vi "recursively populate tree ctl.vi"(8 "error in (no error)":errorcluster, 10 "Object path":string="IndivITX/Test1/SA03008N.20190801.000000.itx", 11 "tree ctl ref":refnum<vi>) -> (0 "error out":errorcluster, 3 "reference out":refnum<vi>)   [LabVIEW 2019, in "LV-Data.S3.lvclass"]
uses:
  LV-Data.S3.lvclass
panel:
  in  "Tree":string(tree)
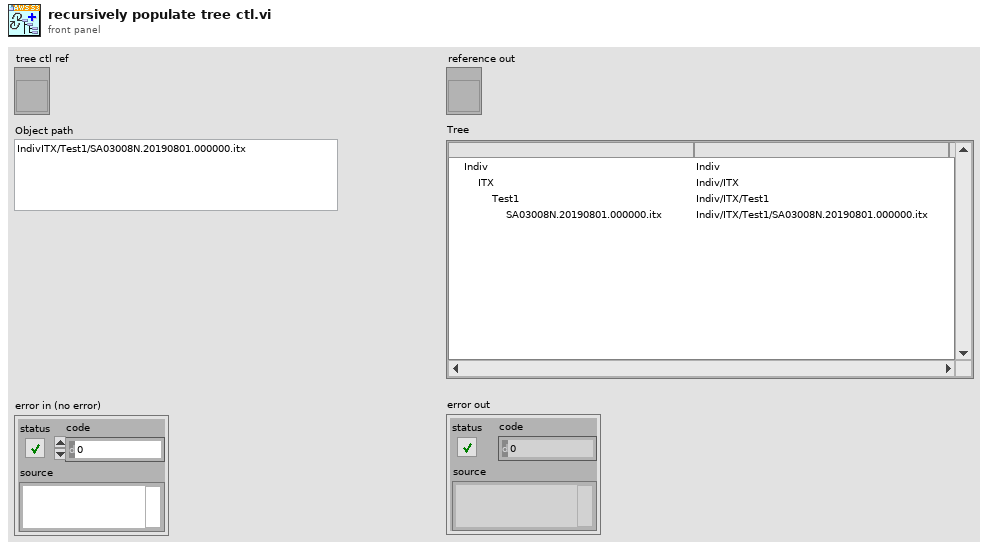
[diagram p1: front panel]
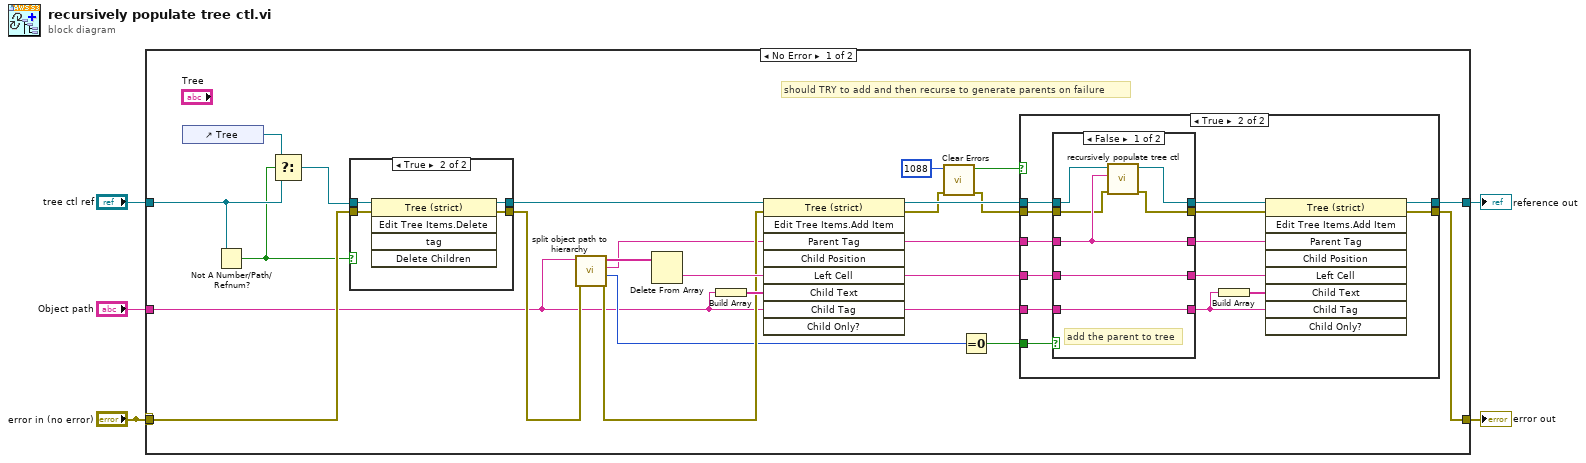
[diagram p0: block diagram]
diagram:
  n1 = case shown="No Error" "error in (no error)" {
    selector: "error in (no error)" -> [_ w62]
    tunnel: [w17 w62] -> w5
    tunnel: [w23 w63] -> w4
    tunnel: "Object path" -> [w8 _]
    tunnel: "tree ctl ref" -> [w7 w63]
    tunnel: "error in (no error)" -> [w10 _]
    frame No Error {
      # "should TRY to add and then recurse to generate parents on failure"
      n2 = control-ref of="Tree"() -> (w18:refnum<vi>)
      n3 = Not A Number/Path/Refnum?(number/path/refnum=w7) -> (NaN/Path/Refnum?=w6:bool)
      n4 = Select(t=w18, s=w6, f=w7) -> (s? t:f=w12:refnum<vi>)
      n5 = case shown="True" w6 {
        tunnel: w12 -> [w29 w33]
        tunnel: [w29 w32] -> w11
        tunnel: w10 -> [w28 w31]
        tunnel: [w28 w30] -> w9
        frame False {
        }
        frame True {
          n6 = invoke class="Tree (strict)" method="Edit Tree Items.Delete"(reference=w33, error in=w31) -> (reference out=w32:refnum<vi>, error out=w30:errorcluster)  [unwired: 3 in, 3 out]
        }
      }
      n7 = call "split object path to hierarchy.vi"("error in (no error)"=w9, "Object path"=w8) -> ("error out"=w19:errorcluster, "layers"=w14:i32, "parent path"=w13:string, "hierarchy"=w21:string[])  [unwired: 6 in]
      n8 = Delete From Array(array=w21) -> (deleted portion=w20:string)  [unwired: 2 in, 1 out]
      n9 = Build Array(w8) -> (w26:string[])
      n10 = invoke on="Invoke Node" class="Tree (strict)" method="Edit Tree Items.Add Item"(reference=w11, error in=w19, "Parent Tag"=w13, "Left Cell"=w20, "Child Text"=w26, "Child Tag"=w8) -> (reference out=w22:refnum<vi>, error out=w16:errorcluster)  [unwired: 3 in, 7 out]
      n11 = call <vilib>:"Clear Errors.vi"("error in (no error)"=w16, "specific error code to clear (0: all)"=1088) -> ("error out"=w15:errorcluster, "specific error cleared?"=w25:bool)  [unwired: 4 in]
      n12 = Equal To 0?(x=w14) -> (x = 0?=w27:bool)
      n13 = case shown="True" w25 {
        tunnel: [w35 w44] -> w17
        tunnel: w27 -> [_ w49]
        tunnel: [w34 w45] -> w23
        tunnel: w15 -> [w35 w48]
        tunnel: w13 -> [_ w42]
        tunnel: w22 -> [w34 w43]
        tunnel: w8 -> [_ w36]
        tunnel: w20 -> [_ w38]
        frame False {
        }
        frame True {
          n14 = case shown="False" w49 {
            tunnel: w48 -> [w51 w61]
            tunnel: w42 -> [w54 w59]
            tunnel: [w50 w61] -> w47
            tunnel: w43 -> [w55 w60]
            tunnel: [w56 w60] -> w46
            tunnel: [w54 w59] -> w40
            tunnel: [w53 w58] -> w39
            tunnel: w38 -> [w53 w58]
            tunnel: [w52 w57] -> w37
            tunnel: w36 -> [w52 w57]
            frame False {
              # "add the parent to tree"
              n15 = call "recursively populate tree ctl.vi"("error in (no error)"=w51, "Object path"=w54, "tree ctl ref"=w55) -> ("error out"=w50:errorcluster, "reference out"=w56:refnum<vi>)  [unwired: 7 in]
            }
            frame True {
            }
          }
          n16 = Build Array(w37) -> (w41:string[])
          n17 = invoke on="Invoke Node" class="Tree (strict)" method="Edit Tree Items.Add Item"(reference=w46, error in=w47, "Parent Tag"=w40, "Left Cell"=w39, "Child Text"=w41, "Child Tag"=w37) -> (reference out=w45:refnum<vi>, error out=w44:errorcluster)  [unwired: 3 in, 7 out]
        }
      }
    }
    frame Error {
    }
  }
  "error out" <- w5
  "reference out" <- w4
